vi "User Console View.vi"(8 "error in (no error)":errorcluster, 11 "View Model":T1) -> (0 "error out":errorcluster)   [LabVIEW 2017]
doc: "This simulated HW Console View. Contains human input."
uses:
  View Model/Controls/View Model.ctl
  Error Handler/Controls/Error Model.ctl
  Error Handler/Controls/Error EventData.ctl
  Error Handler/Controls/Error Type.ctl
  Elevator Controller/Controls/Elevator Model.ctl
  Elevator Controller/Controls/Elevator Overhead.ctl
  Elevator Controller/Controls/Elevator States.ctl
  Elevator Controller/Controls/Elevator Location.ctl
  Elevator Controller/Controls/Elevator Command Event.ctl
  Elevator Controller/Controls/Elevator Commands.ctl
  Configuration/Controls/Configuration Model.ctl
  Configuration/Controls/Configuration Data.ctl
  View Model/Controls/Shared Model.ctl
  Controls/User Console View.ctl
panel:
  in  "Emergency":bool
  in  "1st Floor":bool
  in  "2nd Floor":bool
  in  "3rd Floor":bool
  in  "4th Floor":bool
  in  "Close Door":bool
  in  "Open Door":bool
  in  "Down 4":bool
  in  "Down 3":bool
  in  "Down 2":bool
  in  "Up 3":bool
  in  "Up 2":bool
  in  "Up 1":bool
  # "[Covers: UI1]"
  # "Floor Selection"
  # "Elevator Call"
  # "[Covers UI2A1]"
  # "[Covers: UI2C]"
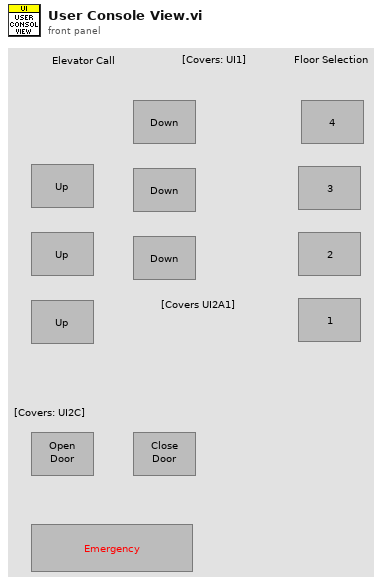
[diagram p1: front panel]
types:
  T1 = typedef "View Model.ctl" = cluster{"Error Model":T2, "Elevator Model":T3, "Configuration Model":T4, "Shared Model":T5}
  T2 = typedef "Error Model.ctl" = cluster{"Error Event":refnum<user-event>}
  T3 = typedef "Elevator Model.ctl" = cluster{"Elevator Overhead":refnum<data-value>, "Floor Change":refnum<user-event>, "Elevator CMD":refnum<user-event>, "Motion Change":refnum<user-event>, "Direction Change":refnum<user-event>, "Door Position Change":refnum<user-event>, "Emergency Change":refnum<user-event>}
  T4 = typedef "Configuration Model.ctl" = cluster{"Config Change":refnum<user-event>, "Config DVR":refnum<data-value>}
  T5 = typedef "Shared Model.ctl" = cluster{"Stop DVR":refnum<data-value>, "Stop Event":refnum<user-event>}
  T6 = typedef "User Console View.ctl" = cluster{"Down 2":refnum<vi>, "Down 3":refnum<vi>, "Down 4":refnum<vi>, "Up 1":refnum<vi>, "Up 2":refnum<vi>, "Up 3":refnum<vi>, "1st Floor":refnum<vi>, "3rd Floor":refnum<vi>, "2nd Floor":refnum<vi>, "4th Floor":refnum<vi>, "Open Door":refnum<vi>, "Close Door":refnum<vi>, "Emergency":refnum<vi>}
  T7 = typedef "Elevator Commands.ctl" = enum16{"Go Up", "Go Down", "Go to Floor", "Emergency", "Open Doors", "Close Doors"}
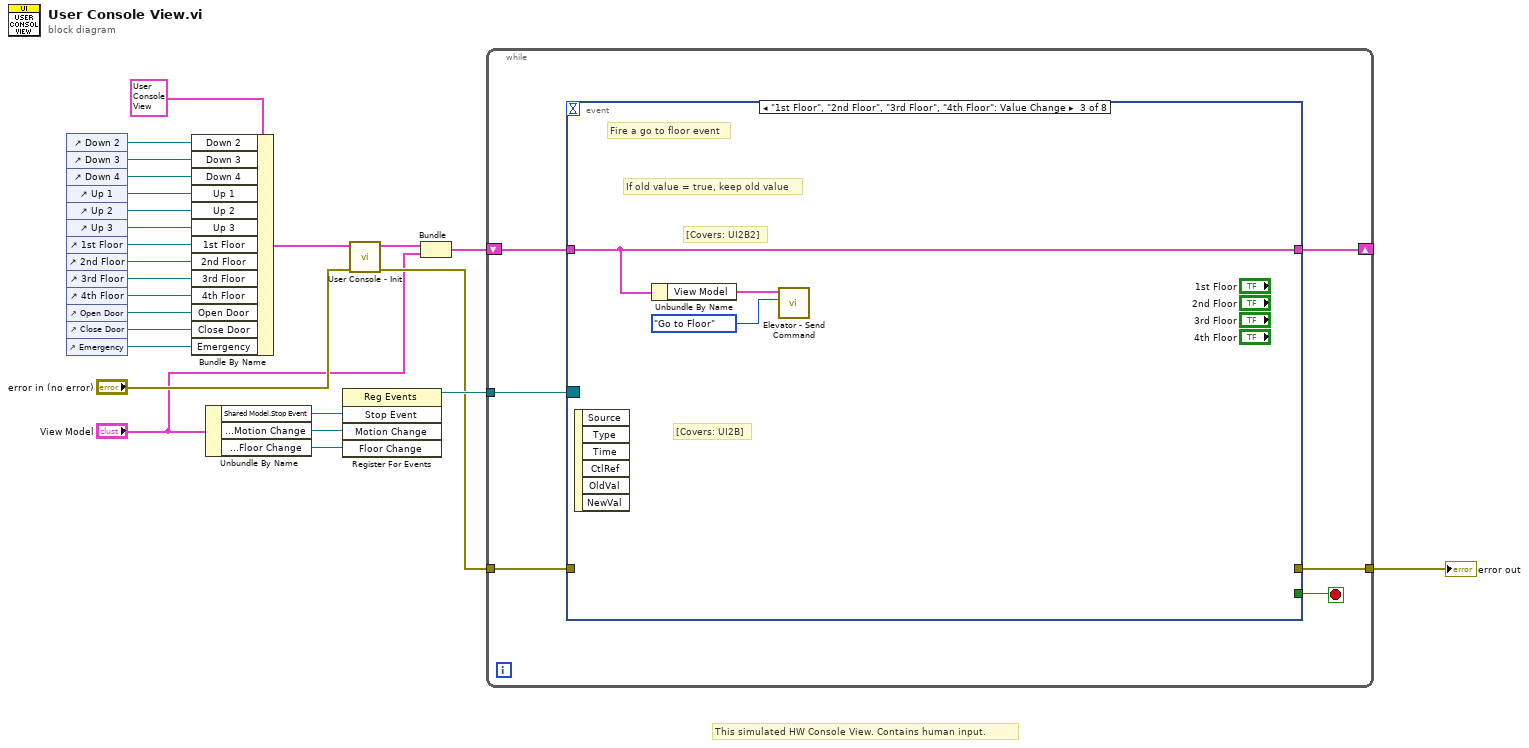
[diagram p0: block diagram]
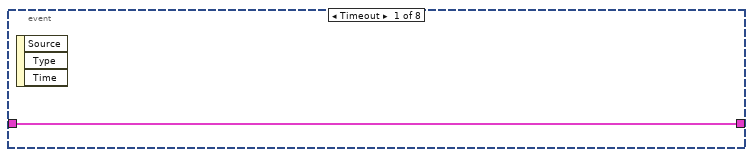
[diagram p2: hidden frame]
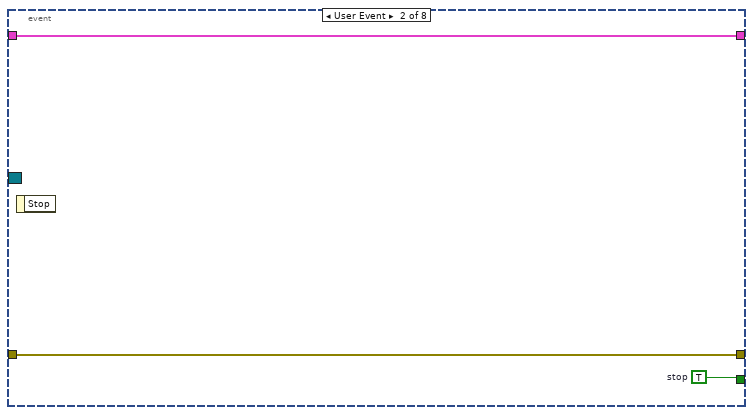
[diagram p3: hidden frame]
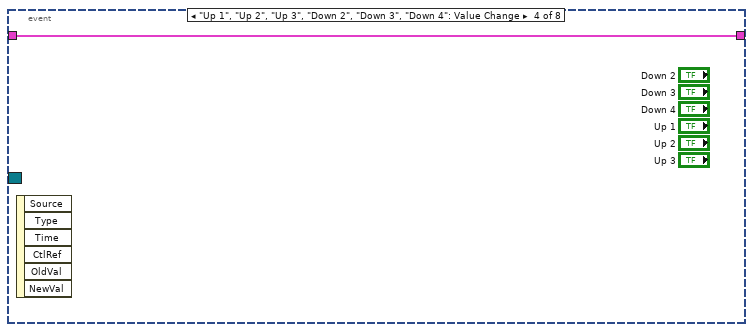
[diagram p4: hidden frame]
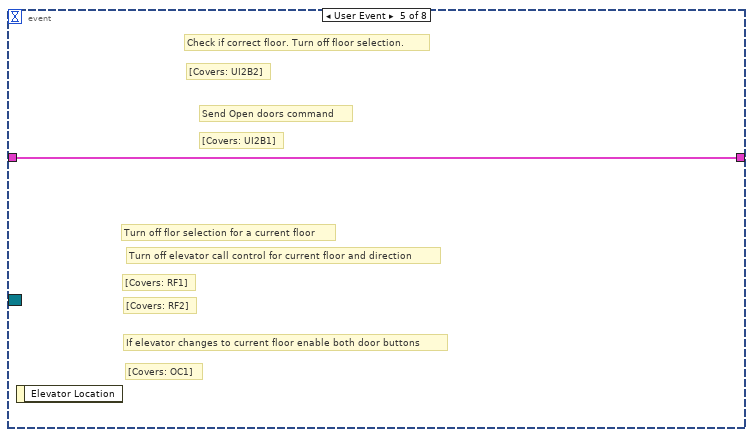
[diagram p5: hidden frame]
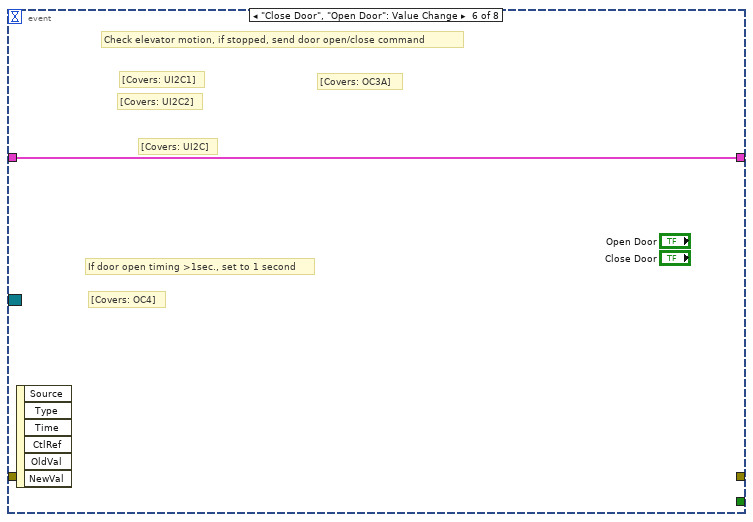
[diagram p6: hidden frame]
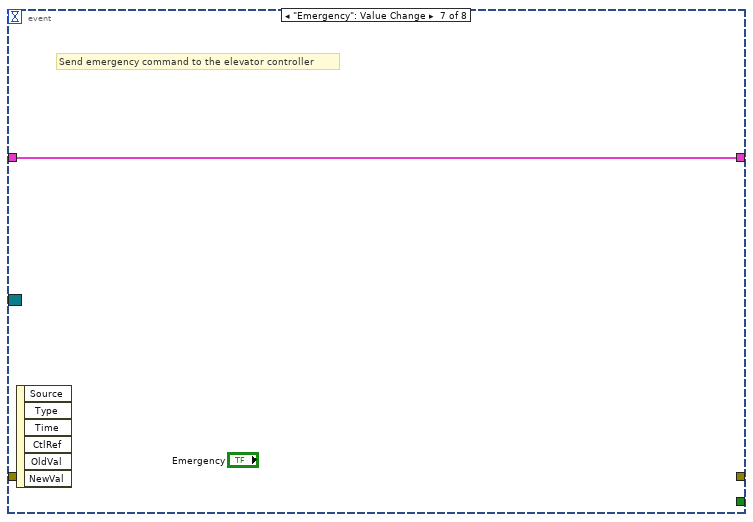
[diagram p7: hidden frame]
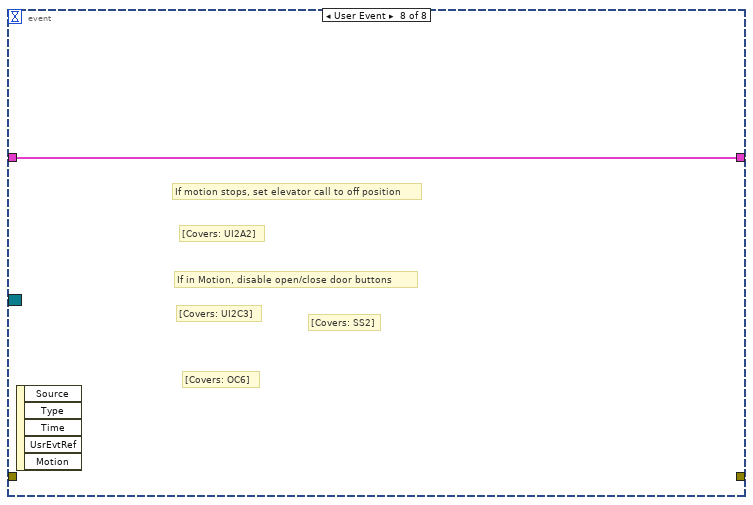
[diagram p8: hidden frame]
diagram:
  # "This simulated HW Console View. Contains human input."
  n1 = control-ref of="Down 2"() -> (w20:refnum<vi>)
  n2 = control-ref of="Down 3"() -> (w18:refnum<vi>)
  n3 = control-ref of="Down 4"() -> (w17:refnum<vi>)
  n4 = control-ref of="Up 1"() -> (w16:refnum<vi>)
  n5 = control-ref of="Up 2"() -> (w15:refnum<vi>)
  n6 = control-ref of="Up 3"() -> (w14:refnum<vi>)
  n7 = control-ref of="1st Floor"() -> (w13:refnum<vi>)
  n8 = control-ref of="2nd Floor"() -> (w12:refnum<vi>)
  n9 = control-ref of="3rd Floor"() -> (w11:refnum<vi>)
  n10 = control-ref of="4th Floor"() -> (w10:refnum<vi>)
  n11 = control-ref of="Open Door"() -> (w9:refnum<vi>)
  n12 = control-ref of="Close Door"() -> (w8:refnum<vi>)
  n13 = control-ref of="Emergency"() -> (w19:refnum<vi>)
  n14 = Bundle By Name(cluster=T6 {"Down 2"=refnum, "Down 3"=refnum, "Down 4"=refnum, "Up 1"=refnum, "Up 2"=refnum, "Up 3"=refnum, "1st Floor"=refnum, "3rd Floor"=refnum, "2nd Floor"=refnum, "4th Floor"=refnum, "Open Door"=refnum, "Close Door"=refnum, "Emergency"=refnum} ("User Console View"), "Down 2"=w20, "Down 3"=w18, "Down 4"=w17, "Up 1"=w16, "Up 2"=w15, "Up 3"=w14, "1st Floor"=w13, "2nd Floor"=w12, "3rd Floor"=w11, "4th Floor"=w10, "Open Door"=w9, "Close Door"=w8, "Emergency"=w19) -> (w6:T6)
  n15 = Unbundle By Name("View Model") -> ("Shared Model.Stop Event"=w25:refnum<user-event>, "Elevator Model.Motion Change"=w24:refnum<user-event>, "Elevator Model.Floor Change"=w7:refnum<user-event>)
  n16 = register-events(w25, w24, w7) -> (reference out=w23:refnum<event-registration>)  [unwired: 2 in, 1 out]
  n17 = call "User Console - Init.vi"("error in (no error)"="error in (no error)", "User Console View"=w6) -> ("error out"=w4:errorcluster, "User Console View"=w3:T6)  [unwired: 8 in]
  n18 = Bundle("User Console View"=w3, "View Model"="View Model") -> (w1:cluster{"User Console View":T6, "View Model":T1})  [unwired: 1 in]
  n19 = while {
    tunnel: w23 -> [w31]
    tunnel: w4 -> [w30]
    tunnel: [w29] -> w22
    shift-right: [w26] -> _
    shift-left: w1 -> [w27]
    stop <- w28 stop-if-true
    n20 = event shown="[2] \"1st Floor\", \"2nd Floor\", \"3rd Floor\", \"4th Floor\": Value Change" {
      selector: w31 -> [_ _ _ _ _ _ _ _]
      dyn-events: _ -> [_ _ _ _ _ _ _ _]
      timeout: _ -> [_ _ _ _ _ _ _ _]
      tunnel: w30 -> [_ w35 _ _ _ _ _ _]
      tunnel: [_ w35 _ _ _ _ _ _] -> w29
      tunnel: [_ w34 _ _ _ _ _ _] -> w28
      tunnel: w27 -> [w32 w33 w38 w39 w40 w41 w42 w43]
      tunnel: [w32 w33 w38 w39 w40 w41 w42 w43] -> w26
      event Timeout {
        n21 = event-data() -> ()  [unwired: 1 in, 3 out]
      }
      event User Event {
        w34 = TRUE  # stop
        n22 = event-data() -> ()  [unwired: 1 in, 1 out]
      }
      event "1st Floor", "2nd Floor", "3rd Floor", "4th Floor": Value Change {
        # "[Covers: UI2B]"
        # "[Covers: UI2B2]"
        # "If old value = true, keep old value"
        # "Fire a go to floor event"
        n23 = event-data() -> ()  [unwired: 1 in, 6 out]
        n24 = Unbundle By Name(w38) -> ("View Model"=w37:T1)
        n25 = call "Elevator - Send Command.vi"("Elevator Commands"=Elevator_Commands."Go to Floor", "View Model"=w37) -> ()  [unwired: 8 in, 2 out]
      }
      event "Up 1", "Up 2", "Up 3", "Down 2", "Down 3", "Down 4": Value Change {
        n26 = event-data() -> ()  [unwired: 1 in, 6 out]
      }
      event User Event {
        # "[Covers: OC1]"
        # "If elevator changes to current floor enable both door buttons"
        # "[Covers: RF2]"
        # "Turn off elevator call control for current floor and direction"
        # "[Covers: RF1]"
        # "Turn off flor selection for a current floor"
        # "[Covers: UI2B1]"
        # "Send Open doors command"
        # "Check if correct floor. Turn off floor selection."
        # "[Covers: UI2B2]"
        n27 = event-data() -> ()  [unwired: 1 in, 1 out]
      }
      event "Close Door", "Open Door": Value Change {
        # "[Covers: OC4]"
        # "If door open timing >1sec., set to 1 second"
        # "[Covers: OC3A]"
        # "[Covers: UI2C]"
        # "[Covers: UI2C2]"
        # "[Covers: UI2C1]"
        # "Check elevator motion, if stopped, send door open/close command"
        n28 = event-data() -> ()  [unwired: 1 in, 6 out]
      }
      event "Emergency": Value Change {
        # "Send emergency command to the elevator controller"
        n29 = event-data() -> ()  [unwired: 1 in, 6 out]
      }
      event User Event {
        # "[Covers: OC6]"
        # "[Covers: SS2]"
        # "[Covers: UI2C3]"
        # "If in Motion, disable open/close door buttons"
        # "[Covers: UI2A2]"
        # "If motion stops, set elevator call to off position"
        n30 = event-data() -> ()  [unwired: 1 in, 5 out]
      }
    }
  }
  "error out" <- w22
